vi "US TOF CM convertor.vi"(3 "Time of flight (uSec) 3":u32, 4 "Time of flight (uSec)":u32, 5 "Time of flight (uSec) 2":u32) -> (0 "Distance (cm) 3":sgl format="%.2f", 1 "Distance (cm)":sgl format="%.2f", 2 "Distance (cm) 2":sgl format="%.2f")   [LabVIEW 2015]
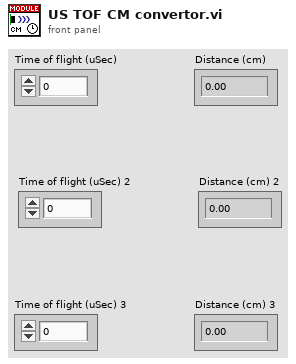
[diagram p1: front panel]
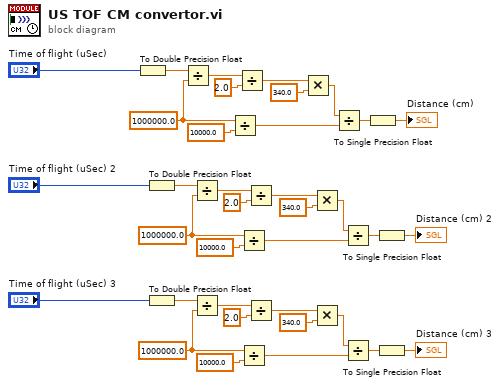
[diagram p0: block diagram]
diagram:
  w8 = 1000000.0 ("y")
  w25 = 1000000.0 ("y")
  w28 = 1000000.0 ("y")
  n1 = To Double Precision Float(number="Time of flight (uSec)") -> (double precision float=w35:dbl)
  n2 = To Double Precision Float(number="Time of flight (uSec) 2") -> (double precision float=w18:dbl)
  n3 = To Double Precision Float(number="Time of flight (uSec) 3") -> (double precision float=w15:dbl)
  n4 = Divide(x=w35, y=w28) -> (x/y=w34:dbl)
  n5 = Divide(x=w18, y=w25) -> (x/y=w19:dbl)
  n6 = Divide(x=w15, y=w8) -> (x/y=w14:dbl)
  n7 = Divide(x=w28, y=10000.0) -> (x/y=w29:dbl)
  n8 = Divide(x=w34, y=2.0) -> (x/y=w32:dbl)
  n9 = Divide(x=w25, y=10000.0) -> (x/y=w24:dbl)
  n10 = Divide(x=w8, y=10000.0) -> (x/y=w9:dbl)
  n11 = Divide(x=w19, y=2.0) -> (x/y=w21:dbl)
  n12 = Divide(x=w14, y=2.0) -> (x/y=w12:dbl)
  n13 = Multiply(x=w32, y=340.0) -> (x*y=w30:dbl)
  n14 = Multiply(x=w21, y=340.0) -> (x*y=w23:dbl)
  n15 = Multiply(x=w12, y=340.0) -> (x*y=w10:dbl)
  n16 = Divide(x=w30, y=w29) -> (x/y=w6:dbl)
  n17 = Divide(x=w23, y=w24) -> (x/y=w5:dbl)
  n18 = Divide(x=w10, y=w9) -> (x/y=w4:dbl)
  n19 = To Single Precision Float(number=w6) -> (single precision float=→"Distance (cm)":sgl)
  n20 = To Single Precision Float(number=w5) -> (single precision float=→"Distance (cm) 2":sgl)
  n21 = To Single Precision Float(number=w4) -> (single precision float=→"Distance (cm) 3":sgl)
